vi "))Channel.vi"(6 "abort (F)":bool, 7 "This VI":refnum<vi>, 8 "element in":T3={"Measurement type"=enum."Debug", "Sensor type"=enum."IFX_8in_256ch", "Identifier"="test.txt", "Open after execution?"=FALSE, "Plot after execution?"=FALSE, "Display channel"=0, "Voltage Delay (s)"=0.5, "Switch Delay (s)"=0.01, "VISA resource name source"="", "VISA resource name DMM"="", "VISA resource name LCR"="", "Compliance  Level (A)"=1e-05, "Voltage Limit (V)"=1000.0, "Data storage location"="", "Scan voltages"="", "Use source as DMM?"=FALSE, "LCR signal frequenzy (Hz)"=10000.0, "DMM device"=enum."Keithley2450", "Sampling number"=1, "Use env. sensors on"=enum."Sensirion sht1x/7x", "Switchboard Handle"=0, "Use Switchboard"=FALSE, "LCR signal voltage (V)"=10000.0, "Repeat"=1, "Scan voltages IV"="", "Scan voltages CV"="", "Hex pad numbers?"=FALSE, "Set measurement type"=enum."Debug", "Custom pad scan"="", "IV voltage Delay (s)"=0.5, "CV voltage Delay (s)"=0.5, "Needle measurement?"=FALSE, "Comments"="test.txt", "LCR signal frequenzy (kHz)"=10.0, "Compliance  Level (uA)"=10.0, "Open Correction Array"=array2304x3[6912 elements], "Current set voltage"=0.0, "Last set voltage"=0.0, "Current channel"=0, "Last OpenCorrection index"=-1, "Total curr/vltg every x steps"=10, "Current channel iteration"=0, "No CV corrections"=FALSE, "Mapfile"="", "Corrfile"="", "IV voltage file"=path "", "CV voltage file"=path "", "IV Switch Delay (s)"=0.01, "CV Switch Delay (s)"=0.01, "Invert polarity"=FALSE, "Set debug dirs"=FALSE, "Is n on p"=FALSE, "Source interlock?"=TRUE, "Voltage file used?"=FALSE, "Pad mask"="", "Mask pad above (uA)"=1.0, "LCR device"=enum."LCR_E4980", "Source device"=enum."Source_2410", "HexPlot binary path"=""} {"CV Switch Delay (s)" format="%#_13g"; "IV Switch Delay (s)" format="%#_13g"; "Last set voltage" format="%#_13g"; "Current set voltage" format="%#_13g"; "CV voltage Delay (s)" format="%#_13g"; "IV voltage Delay (s)" format="%#_13g"; "Voltage Limit (V)" format="%#_13g"; "Voltage Delay (s)" format="%#_13g"; "Switch Delay (s)" format="%#_13g"}, 10 "channelOp":T2=enum."write", 11 "channel in":T1) -> (0 "element out":T3={"Measurement type"=enum."Debug", "Sensor type"=enum."IFX_8in_256ch", "Identifier"="test.txt", "Open after execution?"=FALSE, "Plot after execution?"=FALSE, "Display channel"=0, "Voltage Delay (s)"=0.5, "Switch Delay (s)"=0.01, "VISA resource name source"="", "VISA resource name DMM"="", "VISA resource name LCR"="", "Compliance  Level (A)"=1e-05, "Voltage Limit (V)"=1000.0, "Data storage location"="", "Scan voltages"="", "Use source as DMM?"=FALSE, "LCR signal frequenzy (Hz)"=10000.0, "DMM device"=enum."Keithley2450", "Sampling number"=1, "Use env. sensors on"=enum."Sensirion sht1x/7x", "Switchboard Handle"=0, "Use Switchboard"=FALSE, "LCR signal voltage (V)"=10000.0, "Repeat"=1, "Scan voltages IV"="", "Scan voltages CV"="", "Hex pad numbers?"=FALSE, "Set measurement type"=enum."Debug", "Custom pad scan"="", "IV voltage Delay (s)"=0.5, "CV voltage Delay (s)"=0.5, "Needle measurement?"=FALSE, "Comments"="test.txt", "LCR signal frequenzy (kHz)"=10.0, "Compliance  Level (uA)"=10.0, "Open Correction Array"=array2304x3[6912 elements], "Current set voltage"=0.0, "Last set voltage"=0.0, "Current channel"=0, "Last OpenCorrection index"=-1, "Total curr/vltg every x steps"=10, "Current channel iteration"=0, "No CV corrections"=FALSE, "Mapfile"="", "Corrfile"="", "IV voltage file"=path "", "CV voltage file"=path "", "IV Switch Delay (s)"=0.01, "CV Switch Delay (s)"=0.01, "Invert polarity"=FALSE, "Set debug dirs"=FALSE, "Is n on p"=FALSE, "Source interlock?"=TRUE, "Voltage file used?"=FALSE, "Pad mask"="", "Mask pad above (uA)"=1.0, "LCR device"=enum."LCR_E4980", "Source device"=enum."Source_2410", "HexPlot binary path"=""} {"CV Switch Delay (s)" format="%#_13g"; "IV Switch Delay (s)" format="%#_13g"; "Last set voltage" format="%#_13g"; "Current set voltage" format="%#_13g"; "CV voltage Delay (s)" format="%#_13g"; "IV voltage Delay (s)" format="%#_13g"; "Voltage Limit (V)" format="%#_13g"; "Voltage Delay (s)" format="%#_13g"; "Switch Delay (s)" format="%#_13g"}, 1 "sequence":u64, 2 "wait":refnum<k4>, 3 "channel out":T1, 4 "aborted?":bool, 5 "This VI out":refnum<vi>)   [LabVIEW 2020, in "Tag-t'input_params.ctl'.lvlib"]
uses:
  <extravilib>/ChannelInstances/Tag-t'input_params.ctl'.lvlib
  Desktop/HexDAQ/src/input_params.ctl
  <extravilib>/ChannelInstances/Tag-t'input_params.ctl'/ChannelOp.ctl
  <extravilib>/ChannelInstances/Tag-t'input_params.ctl'/))Channel.ctl
  <extravilib>/ChannelInstances/Tag-t'input_params.ctl'/TagData.lvclass
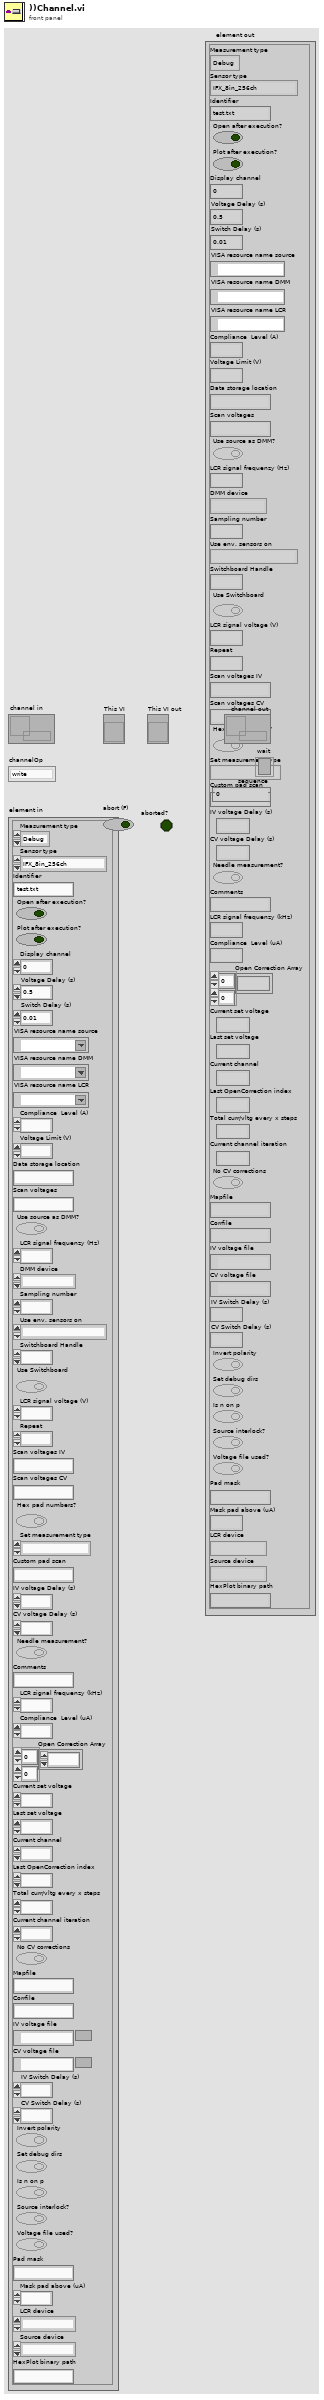
[diagram p1: front panel]
types:
  T1 = typedef "Tag-t'input_params.ctl'.lvlib/))Channel.ctl" = refnum<queue>
  T2 = typedef "Tag-t'input_params.ctl'.lvlib/ChannelOp.ctl" = enum16{"init", "write", "read", "probe"}
  T3 = typedef "input_params.ctl" = cluster{"Measurement type":enum16{"IV", "CV", "Debug", "Test_contact"}, "Sensor type":enum16{"HPK_6in_135ch", "HPK_8in_271ch", "IFX_8in_256ch", "Diode", "HPK_6in_239ch", "Full_Matrix", "HPK_8in_271ch_full", "HPK_8in_198ch", "LumiCal", "HPK_8in_444ch", "HPK_8in_198ch_2019"}, "Identifier":string, "Open after execution?":bool, "Plot after execution?":bool, "Display channel":i32, "Voltage Delay (s)":dbl, "Switch Delay (s)":dbl, "VISA resource name source":refnum<visa-resource-name>, "VISA resource name DMM":refnum<visa-resource-name>, "VISA resource name LCR":refnum<visa-resource-name>, "Compliance  Level (A)":dbl, "Voltage Limit (V)":dbl, "Data storage location":string, "Scan voltages":string, "Use source as DMM?":bool, "LCR signal frequenzy (Hz)":dbl, "DMM device":enum16{"Keithley2001", "Keithley2450", "Keithley2410", "Keithley6485", "Keithley6487", "Keithley6517"}, "Sampling number":i32, "Use env. sensors on":enum16{"Sensirion sht1x/7x", "Switch Matrix", "Probecard"}, "Switchboard Handle":u32, "Use Switchboard":bool, "LCR signal voltage (V)":dbl, "Repeat":i32, "Scan voltages IV":string, "Scan voltages CV":string, "Hex pad numbers?":bool, "Set measurement type":enum16{"IV", "CV", "Debug", "Test_contact", "IV+CV"}, "Custom pad scan":string, "IV voltage Delay (s)":dbl, "CV voltage Delay (s)":dbl, "Needle measurement?":bool, "Comments":string, "LCR signal frequenzy (kHz)":dbl, "Compliance  Level (uA)":dbl, "Open Correction Array":dbl[][], "Current set voltage":dbl, "Last set voltage":dbl, "Current channel":i32, "Last OpenCorrection index":i32, "Total curr/vltg every x steps":i32, "Current channel iteration":i32, "No CV corrections":bool, "Mapfile":string, "Corrfile":string, "IV voltage file":path, "CV voltage file":path, "IV Switch Delay (s)":dbl, "CV Switch Delay (s)":dbl, "Invert polarity":bool, "Set debug dirs":bool, "Is n on p":bool, "Source interlock?":bool, "Voltage file used?":bool, "Pad mask":string, "Mask pad above (uA)":dbl, "LCR device":enum16{"LCR_E4980", "AGILENT_4263X"}, "Source device":enum16{"Source_2410", "Source_6487"}, "HexPlot binary path":string}
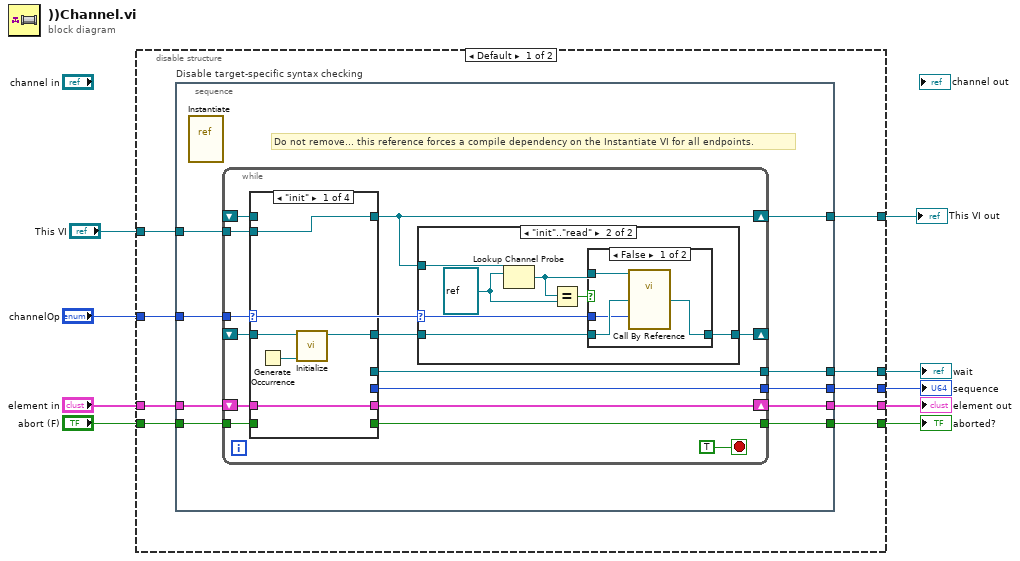
[diagram p0: block diagram]
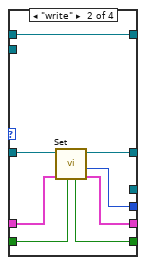
[diagram p2: hidden frame]
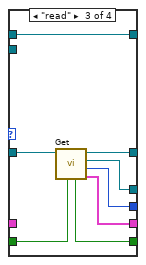
[diagram p3: hidden frame]
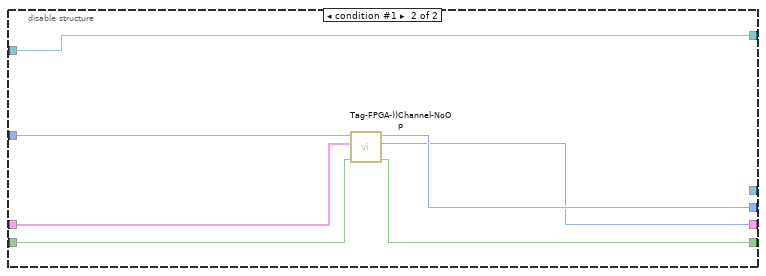
[diagram p7: hidden frame]
diagram:
  n1 = disable-structure "Conditional Disable Structure" shown="Default" {
    disable-tunnel: "channelOp" -> [w17 w85]
    disable-tunnel: "element in" -> [w18 w84]
    disable-tunnel: [w15 w83] -> w7
    disable-tunnel: [w14 w82] -> w6
    disable-tunnel: [w16 _] -> w5
    disable-tunnel: "abort (F)" -> [w13 w81]
    disable-tunnel: [w12 w80] -> w3
    disable-tunnel: "This VI" -> [w11 w79]
    disable-tunnel: [w10 w79] -> w1
    frame condition #0 (active) {
      n2 = stacked-sequence "Disable target-specific syntax checking" {
        tunnel: w18 -> [w27]
        tunnel: w17 -> [w26]
        tunnel: [w25] -> w16
        tunnel: [w24] -> w15
        tunnel: [w23] -> w14
        tunnel: w13 -> [w22]
        tunnel: [w21] -> w12
        tunnel: w11 -> [w20]
        tunnel: [w19] -> w10
        frame #0 {
          # "Do not remove... this reference forces a compile dependency on the Instantiate VI for all endpoints."
          n3 = vi-ref <extravilib>:"Instantiate.vi"() -> ()  [unwired: 1 out]
          n4 = while {
            tunnel: w26 -> [w31]
            shift-right: [w35] -> _
            shift-left: _ -> [w41]
            tunnel: [w39] -> w25
            tunnel: [w38] -> w24
            tunnel: w22 -> [w33]
            tunnel: [w32] -> w21
            shift-right: [w28] -> w19
            shift-left: _ -> [w29]
            tunnel: w20 -> [w30]
            shift-right: [w37] -> w23
            shift-left: w27 -> [w36]
            stop <- TRUE stop-if-true
            n5 = case shown="\"init\"" w31 {
              tunnel: [w46 w53 w61 w65] -> w34
              tunnel: w41 -> [w45 w54 w62 w65]
              tunnel: [_ _ w60 _] -> w39
              tunnel: [_ w51 w59 _] -> w38
              tunnel: [w42 w47 w58 w63] -> w37
              tunnel: w36 -> [w42 w52 _ w63]
              tunnel: w33 -> [_ w50 w56 _]
              tunnel: [_ w49 w57 _] -> w32
              tunnel: w30 -> [w43 _ _ _]
              tunnel: [w43 w48 w55 w64] -> w28
              tunnel: w29 -> [_ w48 w55 w64]
              frame "init" {
                n6 = Generate Occurrence() -> (w44:refnum<k4>)
                n7 = call <extravilib>:"Initialize.vi"("update"=w44, "TagData in"=w45) -> ("TagData out"=w46:refnum<class "TagData.lvclass">)  [unwired: 9 in]
              }
              frame "write" {
                n8 = call <extravilib>:"Set.vi"("abort (F)"=w50, "element"=w52, "TagData in"=w54) -> ("previous element"=w47:T3, "sequence"=w51:u64, "TagData out"=w53:refnum<class "TagData.lvclass">, "aborted?"=w49:bool)  [unwired: 5 in]
              }
              frame "read" {
                n9 = call <extravilib>:"Get.vi"("abort (F)"=w56, "TagData in"=w62) -> ("element"=w58:T3, "sequence"=w59:u64, "update"=w60:refnum<k4>, "TagData out"=w61:refnum<class "TagData.lvclass">, "aborted?"=w57:bool)  [unwired: 5 in]
              }
              frame "probe" {
              }
            }
            n10 = case shown="\"init\"..\"read\"" w31 {
              selector: w31 -> [_ w69]
              tunnel: w34 -> [w66 w71]
              tunnel: [w66 w70] -> w35
              tunnel: w28 -> [_ w67]
              frame Default {
              }
              frame "init".."read" {
                w68 = refnum<vi> refnum ("This VI")
                n11 = Lookup Channel Probe(0:w67, 1:w68) -> (9:w72:refnum<vi>)  [unwired: 1 in, 1 out]
                n12 = Equal?(x=w72, y=w68) -> (x = y?=w73:bool)
                n13 = case shown="False" w73 {
                  tunnel: w72 -> [w77 _]
                  tunnel: w71 -> [w76 w78]
                  tunnel: [w75 w78] -> w70
                  tunnel: w69 -> [w74 _]
                  frame False {
                    n14 = call-by-ref "?"(reference=w77, "channelOp"=w74, "tagData in"=w76) -> ("tagData out"=w75:refnum<class "TagData.lvclass">)  [unwired: 2 in, 2 out]
                  }
                  frame True {
                  }
                }
              }
            }
          }
        }
      }
    }
    frame condition #1 {
      n15 = call <extravilib>:"Tag-FPGA-))Channel-NoOp.vi"("abort (F)"=w81, "element in"=w84, "channelOp"=w85) -> ("aborted?"=w80:bool, "element out"=w82:i32, "sequence"=w83:i16)  [unwired: 6 in]
    }
  }
  "element out" <- w6
  "wait" <- w5
  "sequence" <- w7
  "aborted?" <- w3
  "This VI out" <- w1
